vi "CreateNewStringWithJitSubstitute.vi"(0 "Subject":string, 1 "CompileOptions":u32 format="%.0x", 2 "pCompileContext":u64 format="%.0x", 3 "JitCompileOptions":u32 format="%.0x", 5 "search pattern":string, 7 "Replacement":string, 9 "Offset":u64, 11 "error in":errorcluster, 12 "MatchOptions":u32 format="%.0x", 13 "pMatchContext":u64 format="%.0x") -> (4 "OutString":string, 15 "error out":errorcluster)   [LabVIEW 2021, in "libpcre2-8.lvlib"]
uses:
  libpcre2-8.lvlib
  Pcre2CompileError.vi
  Pcre2FnkCallError.vi
  Pcre2ErrorNull.vi
  Pcre2LibError.vi
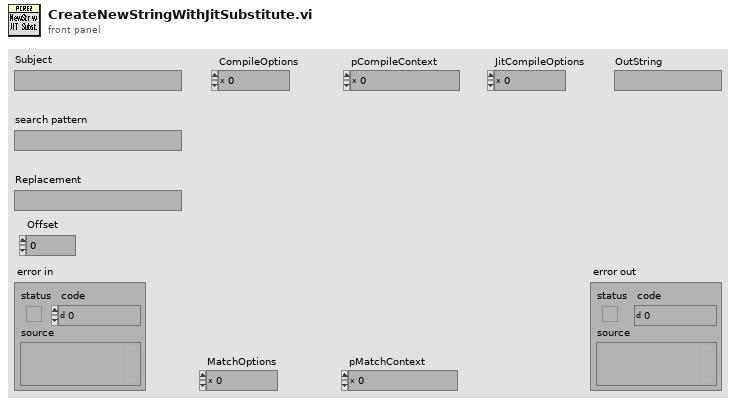
[diagram p1: front panel]
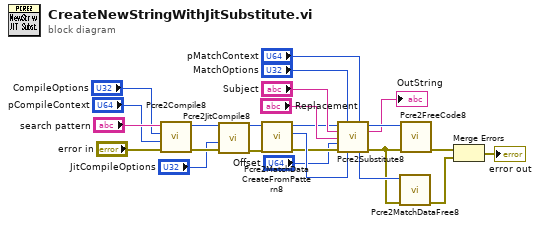
[diagram p0: block diagram]
diagram:
  n1 = call "Pcre2Compile8.vi"("error in"="error in", "pCompileContext"="pCompileContext", "Options"="CompileOptions", "Pattern"="search pattern") -> ("error out"=w4:errorcluster, "pCode"=w5:u64)  [unwired: 6 in]
  n2 = call "Pcre2JitCompile8.vi"("error in"=w4, "Options (1)"="JitCompileOptions", "pCode"=w5) -> ("error out"=w3:errorcluster, "pCode"=w2:u64)  [unwired: 7 in]
  n3 = call "Pcre2MatchDataCreateFromPattern8.vi"("error in"=w3, "pCode"=w2) -> ("error out"=w18:errorcluster, "pMatchData"=w19:u64, "pCode"=w12:u64)  [unwired: 7 in]
  n4 = call "Pcre2Substitute8.vi"("pCode"=w12, "Options"="MatchOptions", "pMatchContext"="pMatchContext", "Subject"="Subject", "Replacement"="Replacement", "StartOffset"="Offset", "error in"=w18, "pMatchData"=w19) -> ("pCode"=w13:u64, "OutString"=→"OutString":string, "pMatchData"=w14:u64, "error out"=w10:errorcluster)  [unwired: 4 in]
  n5 = call "Pcre2MatchDataFree8.vi"("error in"=w10, "pMatchData"=w14) -> ("error out"=w7:errorcluster)  [unwired: 9 in]
  n6 = call "Pcre2FreeCode8.vi"("error in"=w10, "pCode"=w13) -> ("error out"=w9:errorcluster)  [unwired: 9 in]
  n7 = Merge Errors(w9, w7) -> (→"error out":errorcluster)
